vi "FPGA_PPG_set_mode.vi"(0 "resource_in":refnum<visa-resource-name>, 2 "mode":u8(ring) items=["once", "continous"], 5 "error in (no error)":errorcluster) -> (14 "resource_out":refnum<visa-resource-name>, 19 "error out":errorcluster)   [LabVIEW 2014, in "NI-FPGA_PPG_Driver.lvlib"]
doc: "Sets the execution mode of the FPGA (Single run = 0, Continuous = 1).\n\nContact: Falk Ziegler, eMail: ziegler@physik.uni-greifswald.de"
uses:
  NI-FPGA_PPG_Driver.lvlib
  FPGA_PPG_action_type.ctl
  <vilib>/Utility/error.llb/Error Cluster From Error Code.vi
  <vilib>/rvi/errors/niLvFpgaAdjustHostInterfaceError.vi
  <vilib>/rvi/interface/nirviReadWriteControl/nirviReadWriteControl.xnode
  FPGA_PPG_vi_ref.ctl
  FPGA Bitfiles/TiTaProj_COF_PPG_80MHz.lvbitx
  NiFpgaLv.dll
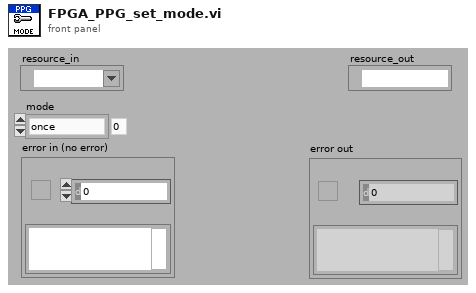
[diagram p1: front panel]
types:
  T1 = typedef "NI-FPGA_PPG_Driver.lvlib/FPGA_PPG_action_type.ctl" = enum16{"GET", "SET", "REMOVE"}
  T2 = typedef "NI-FPGA_PPG_Driver.lvlib/FPGA_PPG_vi_ref.ctl" = refnum<k20>
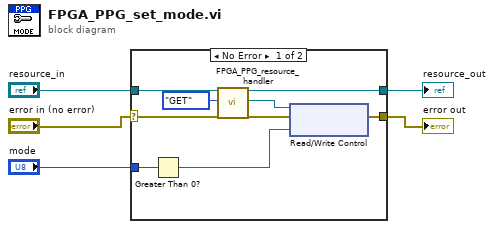
[diagram p0: block diagram]
diagram:
  n1 = case shown="No Error" "error in (no error)" {
    selector: "error in (no error)" -> [w13 w16]
    tunnel: [w8 w16] -> w4
    tunnel: "resource_in" -> [w14 w15]
    tunnel: [w9 w15] -> w2
    tunnel: "mode" -> [w11 _]
    frame No Error {
      n2 = Greater Than 0?(x=w11) -> (x > 0?=w10:bool)
      n3 = call "FPGA_PPG_resource_handler.vi"("resource_in"=w14, "action"=FPGA_PPG_action_type."GET", "error in (no error)"=w13) -> ("resource_out"=w9:refnum<visa-resource-name>, "FPGA VI Reference Out"=w7:T2, "error out"=w12:errorcluster)  [unwired: 14 in]
      n4 = xnode "Read/Write Control"("FPGA VI Reference In"=w7, "error in"=w12, "continuous"=w10) -> ("error out"=w8:errorcluster)  [unwired: 1 out]
    }
    frame Error {
    }
  }
  "error out" <- w4
  "resource_out" <- w2
